vi "Format Value.vi"(4 "Value":dbl format="%#_3f") -> (7 "String":string)   [LabVIEW 2020, in "VolatusGUIElements.lvlib" / "BluelinesRedlines.lvclass"]
uses:
  BluelinesRedlines.lvclass
  BluelinesRedlines.lvclass/BluelinesRedlines.ctl
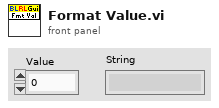
[diagram p1: front panel]
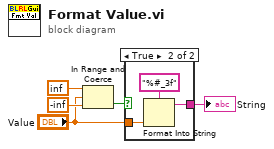
[diagram p0: block diagram]
diagram:
  n1 = In Range and Coerce(upper limit=inf, x="Value", lower limit=-inf) -> (In Range?=w3:bool)  [unwired: 1 out]
  n2 = case shown="True" w3 {
    tunnel: "Value" -> [_ w8]
    tunnel: [_ w6] -> w1
    frame False {
    }
    frame True {
      n3 = Format Into String(format string="%#_3f", w8) -> (resulting string=w6:string)  [unwired: 2 in, 1 out]
    }
  }
  "String" <- w1
